vi "save_2d_array.vi"() -> ()   [LabVIEW 2019]
panel:
  out "selected path":path
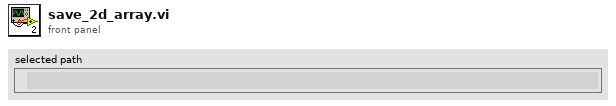
[diagram p1: front panel]
types:
  T1 = enum16{"open", "replace", "create", "open or create", "replace or create", "replace or create with confirmation"}
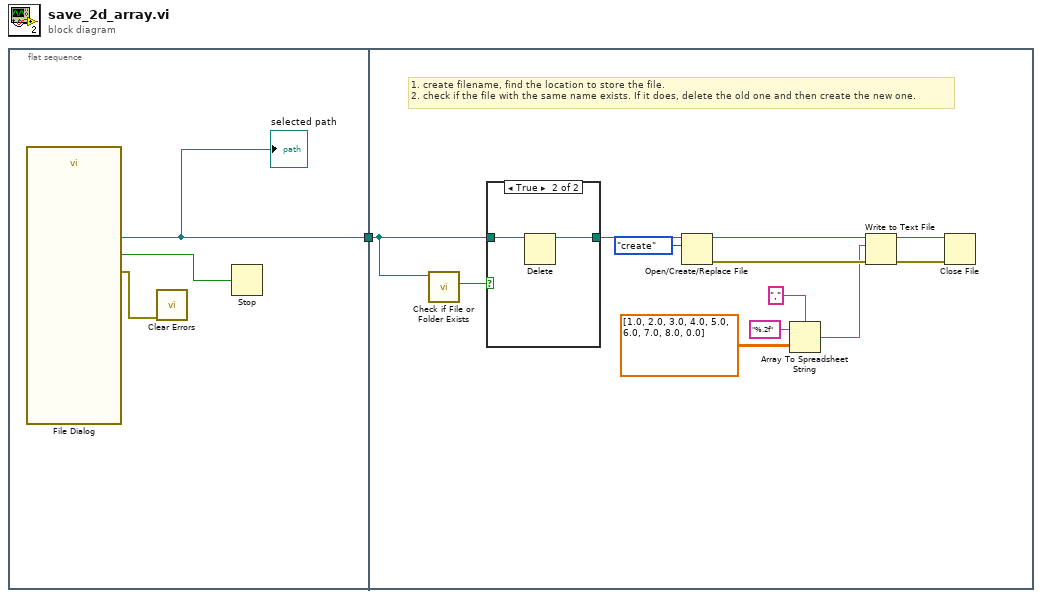
[diagram p0: block diagram]
diagram:
  n1 = flat-sequence {
    tunnel: [w2] -> w1
    tunnel: w1 -> [w15]
    frame #0 {
      n2 = call "File Dialog"() -> ("selected path"=w2:path, "cancelled"=w3:bool, "error out"=w4:errorcluster)  [unwired: 12 in, 1 out]
      "selected path" <- w2
      n3 = call <vilib>:"Clear Errors.vi"("error in (no error)"=w4) -> ()  [unwired: 5 in, 2 out]
      n4 = Stop(stop? (T)=w3) -> ()
    }
    frame #1 {
      # "1. create filename, find the location to store the file.\n2. check if the file with the same name exists. If it does, delete the old one and then create the new one."
      n5 = call <vilib>:"Check if File or Folder Exists.vi"("path"=w15) -> ("file or folder exists?"=w16:bool)  [unwired: 8 in, 2 out]
      n6 = case shown="True" w16 {
        tunnel: w15 -> [w17 w19]
        tunnel: [w17 w18] -> w14
        frame False {
        }
        frame True {
          n7 = Delete(path (use dialog)=w19) -> (deleted path=w18:path)  [unwired: 4 in, 2 out]
        }
      }
      n8 = Open/Create/Replace File(file path (use dialog)=w14, operation (0:open)=T1."create") -> (refnum out=w12:refnum<file>, error out=w11:errorcluster)  [unwired: 4 in, 1 out]
      n9 = Array To Spreadsheet String(delimiter (Tab)=",", array=dbl[][] [[1.0, 2.0, 3.0], [4.0, 5.0, 6.0], [7.0, 8.0, 0.0]], 3:"%.2f" ("format string")) -> (spreadsheet string=w7:string)
      n10 = Write to Text File(file (use dialog)=w12, text=w7, error in=w11) -> (refnum out=w6:refnum<file>, error out=w5:errorcluster)  [unwired: 1 in, 1 out]
      n11 = Close File(refnum=w6, error in=w5) -> ()  [unwired: 2 out]
    }
  }
